vi "CH_LUT.vi"(0 "file path (dialog if empty)":path, 1 "Input#":i32, 3 "Differential\nMode":bool, 9 "Channel LUT IN":string[][](table), 12 "Channel":i32) -> (4 "Ch name":string, 6 "found?":bool, 10 "Channel LUT":string[][](table)=[["1", "1", "Ch0"], ["1", "2", "CH95"], ["1", "3", "Ch1"], ["1", "4", "CH96"], ["1", "5", "CH2"], ["1", "6", "CH97"], ["1", "7", "CH3"], ["1", "8", "CH98"], ["1", "9", "CH4"], ["1", "10", "CH99"], ["1", "11", "CH5"], ["1", "12", "CH100"], ["1", "13", "CH6"], ["1", "14", "CH101"], ["1", "15", "CH7"], ["1", "16", "CH102"], ["2", "1", "CH8"], ["2", "2", "CH103"], ["2", "3", "CH9"], ["2", "4", "CH104"], ["2", "5", "CH10"], ["2", "6", "CH105"], ["2", "7", "CH11"], ["2", "8", "CH106"], ["12", "15", "CH194"], ["2", "9", "CH12"], ["2", "10", "CH107"], ["2", "11", "CH13"], ["2", "12", "CH108"], ["2", "13", "CH14"], ["2", "14", "CH109"], ["2", "15", "CH15"], ["2", "16", "CH110"], ["3", "1", "CH16"], ["3", "2", "CH111"], ["3", "3", "CH17"], ["3", "4", "CH112"], ["3", "5", "CH18"], ["3", "6", "CH113"], ["3", "7", "CH19"], ["3", "8", "CH114"], ["3", "9", "CH20"], ["3", "10", "CH115"], ["3", "11", "CH21"], ["3", "12", "CH116"], ["3", "13", "CH22"], ["3", "14", "CH117"], ["3", "15", "CH23"], ["3", "16", "CH118"], ["4", "1", "CH36"], ["4", "2", "CH131"], ["4", "3", "CH37"], ["4", "4", "CH132"], ["4", "5", "CH38"], ["4", "6", "CH133"], ["4", "7", "CH39"], ["4", "8", "CH134"], ["4", "9", "CH40"], ["4", "10", "CH135"], ["4", "11", "CH41"], ["4", "12", "CH136"], ["4", "13", "CH42"], ["4", "14", "CH137"], ["4", "15", "CH43"], ["4", "16", "CH138"], ["5", "1", "CH44"], ["5", "2", "CH139"], ["5", "3", "CH45"], ["5", "4", "CH140"], ["5", "5", "CH46"], ["5", "6", "CH141"], ["5", "7", "CH47"], ["5", "8", "CH142"], ["12", "16", "CH191"], ["5", "9", "CH24"], ["5", "10", "CH119"], ["5", "11", "CH25"], ["5", "12", "CH120"], ["5", "13", "CH26"], ["5", "14", "CH121"], ["5", "15", "CH27"], ["5", "16", "CH122"], ["6", "1", "CH28"], ["6", "2", "CH123"], ["6", "3", "CH29"], ["6", "4", "CH124"], ["6", "5", "CH30"], ["6", "6", "CH125"], ["6", "7", "CH31"], ["6", "8", "CH126"], ["6", "9", "CH32"], ["6", "10", "CH127"], ["6", "11", "CH33"], ["6", "12", "CH128"], ["6", "13", "CH34"], ["6", "14", "CH129"], ["6", "15", "CH35"], ["6", "16", "CH130"], ["7", "1", "CH48"], ["7", "2", "CH143"], ["7", "3", "CH49"], ["7", "4", "CH144"], ["7", "5", "CH50"], ["7", "6", "CH145"], ["7", "7", "CH51"], ["7", "8", "CH146"], ["7", "9", "CH52"], ["7", "10", "CH147"], ["7", "11", "CH53"], ["7", "12", "CH148"], ["7", "13", "CH54"], ["7", "14", "CH149"], ["7", "15", "CH55"], ["7", "16", "CH150"], ["8", "1", "CH56"], ["8", "2", "CH151"], ["8", "3", "CH57"], ["8", "4", "CH152"], ["8", "5", "CH58"], ["8", "6", "CH153"], ["8", "7", "CH59"], ["8", "8", "CH154"], ["8", "9", "CH60"], ["8", "10", "CH155"], ["8", "11", "CH61"], ["8", "12", "CH156"], ["8", "13", "CH62"], ["8", "14", "CH157"], ["8", "15", "CH63"], ["8", "16", "CH158"], ["9", "1", "CH64"], ["9", "2", "CH159"], ["9", "3", "CH65"], ["9", "4", "CH160"], ["9", "5", "CH66"], ["9", "6", "CH161"], ["9", "7", "CH67"], ["9", "8", "CH162"], ["9", "9", "CH68"], ["9", "10", "CH163"], ["9", "11", "CH69"], ["9", "12", "CH164"], ["9", "13", "CH70"], ["9", "14", "CH165"], ["9", "15", "CH71"], ["9", "16", "CH166"], ["10", "1", "CH84"], ["10", "2", "CH179"], ["10", "3", "CH85"], ["10", "4", "CH180"], ["10", "5", "CH86"], ["10", "6", "CH181"], ["10", "7", "CH87"], ["10", "8", "CH182"], ["10", "9", "CH88"], ["10", "10", "CH183"], ["10", "11", "CH89"], ["10", "12", "CH184"], ["10", "13", "CH90"], ["10", "14", "CH185"], ["10", "15", "CH91"], ["10", "16", "CH186"], ["11", "1", "CH92"], ["11", "2", "CH187"], ["11", "3", "CH93"], ["11", "4", "CH188"], ["11", "5", "CH94"], ["11", "6", "CH189"], ["11", "7", "CH72"], ["11", "8", "CH167"], ["11", "9", "CH73"], ["11", "10", "CH168"], ["11", "11", "CH74"], ["11", "12", "CH169"], ["11", "13", "CH75"], ["11", "14", "CH170"], ["11", "15", "CH76"], ["11", "16", "CH171"], ["12", "1", "CH77"], ["12", "2", "CH172"], ["12", "3", "CH78"], ["12", "4", "CH173"], ["12", "5", "CH79"], ["12", "6", "CH174"], ["12", "7", "CH80"], ["12", "8", "CH175"], ["12", "9", "CH81"], ["12", "10", "CH176"], ["12", "11", "CH82"], ["12", "12", "CH177"], ["12", "13", "CH83"], ["12", "14", "CH178"]], 13 "Negative pair name":string, 14 "Positive pair name":string)   [LabVIEW 2013]
uses:
  <vilib>/Utility/file.llb/Read From Spreadsheet File (string).vi
panel:
  # "Correllate between input no. and CH no."
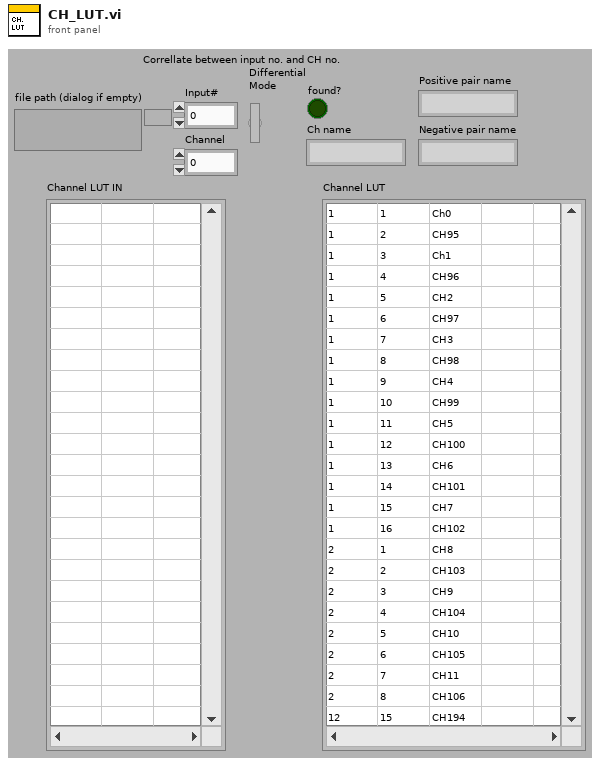
[diagram p1: front panel]
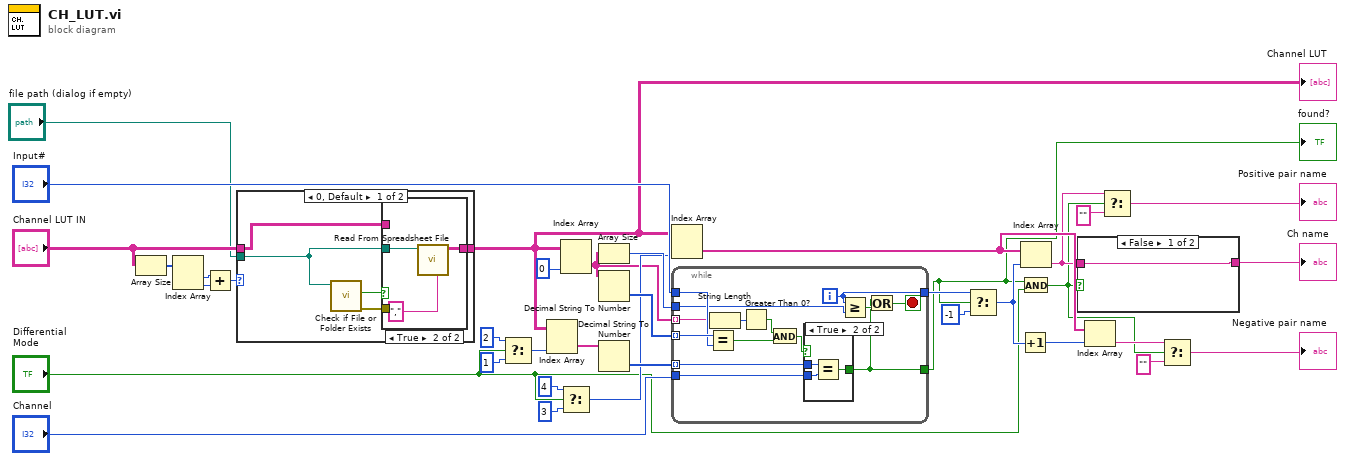
[diagram p0: block diagram]
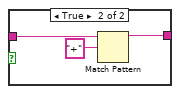
[diagram p2: hidden frame]
diagram:
  n1 = Array Size(array="Channel LUT IN") -> (size(s)=w26:i32[])
  n2 = Index Array(array=w26) -> (element #1=w25:i32, element #2=w24:i32)  [unwired: 2 in]
  n3 = Add(x=w25, y=w24) -> (x+y=w23:i32)
  n4 = case shown="0, Default" w23 {
    tunnel: [w41 w46] -> w30
    tunnel: "Channel LUT IN" -> [w38 w46]
    tunnel: "file path (dialog if empty)" -> [w37 _]
    frame 0, Default {
      n5 = call <vilib>:"Check if File or Folder Exists.vi"("path"=w37) -> ("error out"=w39:errorcluster, "file or folder exists?"=w40:bool)  [unwired: 8 in, 1 out]
      n6 = case shown="True" w40 {
        tunnel: [w42 w44] -> w41
        tunnel: w37 -> [_ w43]
        tunnel: w39 -> [_ _]
        tunnel: w38 -> [w42 _]
        frame False {
        }
        frame True {
          n7 = call-poly <vilib>:"Read From Spreadsheet File.vi"("delimiter (\\t)"="," ("delimiter (\\t)"), "file path (dialog if empty)"=w43) -> ("all rows"=w44:string[][])  [unwired: 5 in, 4 out]
        }
      }
    }
    frame 1.. {
    }
  }
  "Channel LUT" <- w30
  n8 = Select(t=2, s="Differential\nMode", f=1 ("disabled index (col)")) -> (s? t:f=w19:i32)
  n9 = Index Array(array=w30, index (col)=w19) -> (element=w33:string[])  [unwired: 1 in]
  n10 = Index Array(array=w30, index (col)=0 ("disabled index (col)")) -> (element=w15:string[])  [unwired: 1 in]
  n11 = Select(t=4, s="Differential\nMode", f=3 ("t")) -> (s? t:f=w16:i32)
  n12 = Array Size(array=w15) -> (size(s)=w29:i32)
  n13 = Decimal String To Number(string=w15) -> (number=w35:i32[])  [unwired: 2 in, 1 out]
  n14 = Decimal String To Number(string=w33) -> (number=w32:i32[])  [unwired: 2 in, 1 out]
  n15 = Index Array(array=w30, index (col)=w16) -> (element=w12:string[])  [unwired: 1 in]
  n16 = while {
    tunnel: w35 -> [w60] mode=indexing
    tunnel: "Input#" -> [w59]
    tunnel: w32 -> [w58] mode=indexing
    tunnel: "Channel" -> [w57]
    tunnel: [w51] -> w28
    tunnel: [w53] -> w10
    tunnel: w29 -> [w55]
    tunnel: w15 -> [w50] mode=indexing
    i -> [w51]
    stop <- w52 stop-if-true
    n17 = Equal?(x=w60, y=w59) -> (x = y?=w56:bool)
    n18 = String Length(string=w50) -> (length=w49:i32)
    n19 = Greater Than 0?(x=w49) -> (x > 0?=w47:bool)
    n20 = And(x=w47, y=w56) -> (x .and. y?=w48:bool)
    n21 = case shown="True" w48 {
      tunnel: w58 -> [_ w62]
      tunnel: w57 -> [_ w63]
      tunnel: [_ w61] -> w53
      frame False {
      }
      frame True {
        n22 = Equal?(x=w62, y=w63) -> (x = y?=w61:bool)
      }
    }
    n23 = Greater Or Equal?(x=w51, y=w55) -> (x >= y?=w54:bool)
    n24 = Or(x=w53, y=w54) -> (x .or. y?=w52:bool)
  }
  "found?" <- w10
  n25 = Select(t=w28, s=w10, f=-1) -> (s? t:f=w13:i32)
  n26 = Increment(x=w13) -> (x+1=w14:i32)
  n27 = Index Array(array=w12, index=w13) -> (element=w5:string)
  n28 = And(x=w10, y="Differential\nMode") -> (x .and. y?=w4:bool)
  n29 = case shown="False" w4 {
    tunnel: w5 -> [w64 w67]
    tunnel: [w64 w65] -> w6
    frame False {
    }
    frame True {
      n30 = Match Pattern(string=w67, regular expression="+") -> (before substring=w65:string)  [unwired: 1 in, 3 out]
    }
  }
  "Ch name" <- w6
  n31 = Index Array(array=w12, index=w14) -> (element=w8:string)
  n32 = Select(t=w5, s=w4, f="" ("t")) -> (s? t:f=→"Positive pair name":string)
  n33 = Select(t=w8, s=w4, f="" ("t")) -> (s? t:f=→"Negative pair name":string)
